vi "Example_HVI_TDC_DualHistograms.vi"() -> ()   [LabVIEW 2013]
panel:
  out "VI Path":string
  out "cycle Count":i32
  out "Waiting HVI...":i32
  out "Var10=>\nHVIrunning":i32
  in  "Number variable\nHVI runinng":i32=10
  out "Get HVI-Module Status":errorcluster
  out "HVI open Status":errorcluster
  out "errorOut HistogramRead":errorcluster
  in  "bins":i32=50 min=0 max=990 step=10
  out "Histogram":u32[](graph)
  out "histogramOut":u32[](array[numeric])
  in  "Finish Program":bool
  out "Histogram 1 PeakBin":i32
  out "Histogram 1 Peak":i32
  out "Histogram 0 PeakBin":i32
  out "Histogram 0 Peak":i32
  out "Ch1 RateCounter":i32
  out "Ch0 RateCounter":i32
  in  "Number variable \nHistogram 1 PeakBin":i32=5
  in  "Number variable\nHistogram 1 Peak":i32=4
  in  "Number variable \nHistogram 0 PeakBin":i32=3
  in  "Number variable \nHistogram 0 Peak":i32=2
  in  "Name variable \nCh1 RateCounter":string="Variable 1"
  in  "Name variable  \nCh0 RateCounter":string="Variable 0"
  in  "Module name in HVI":string="TDC"
  out "HVIIDOut":i32
  out "moduleIDOut":i32
  out "Close HVI Status":errorcluster
  in  "HVI file":string=".\\Example_HVI_TDC_DualHistograms.HVI"
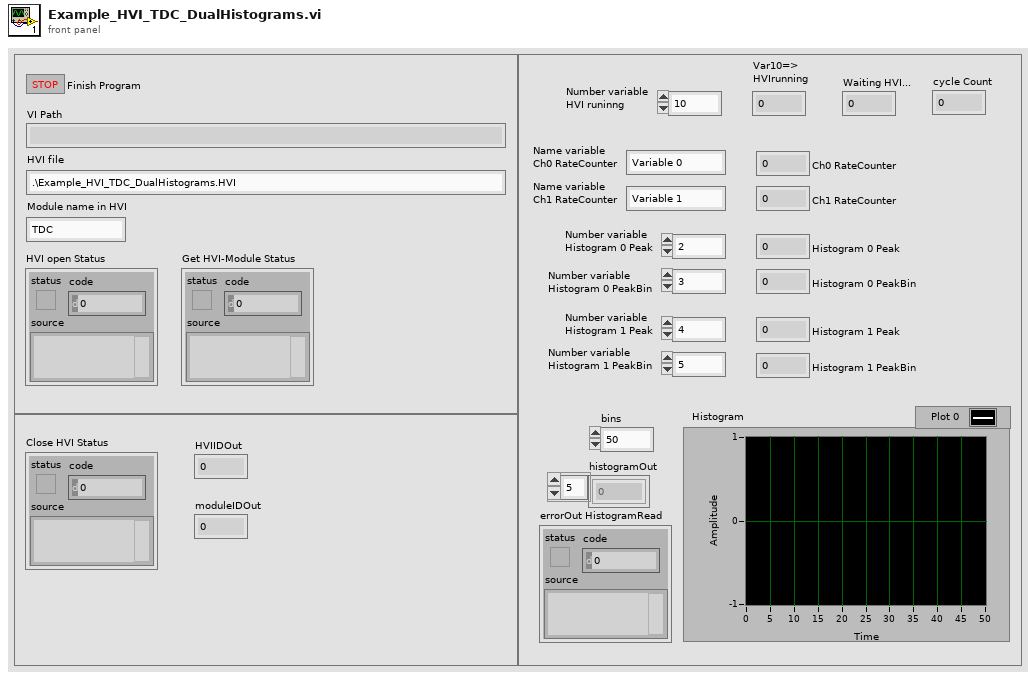
[diagram p1: front panel]
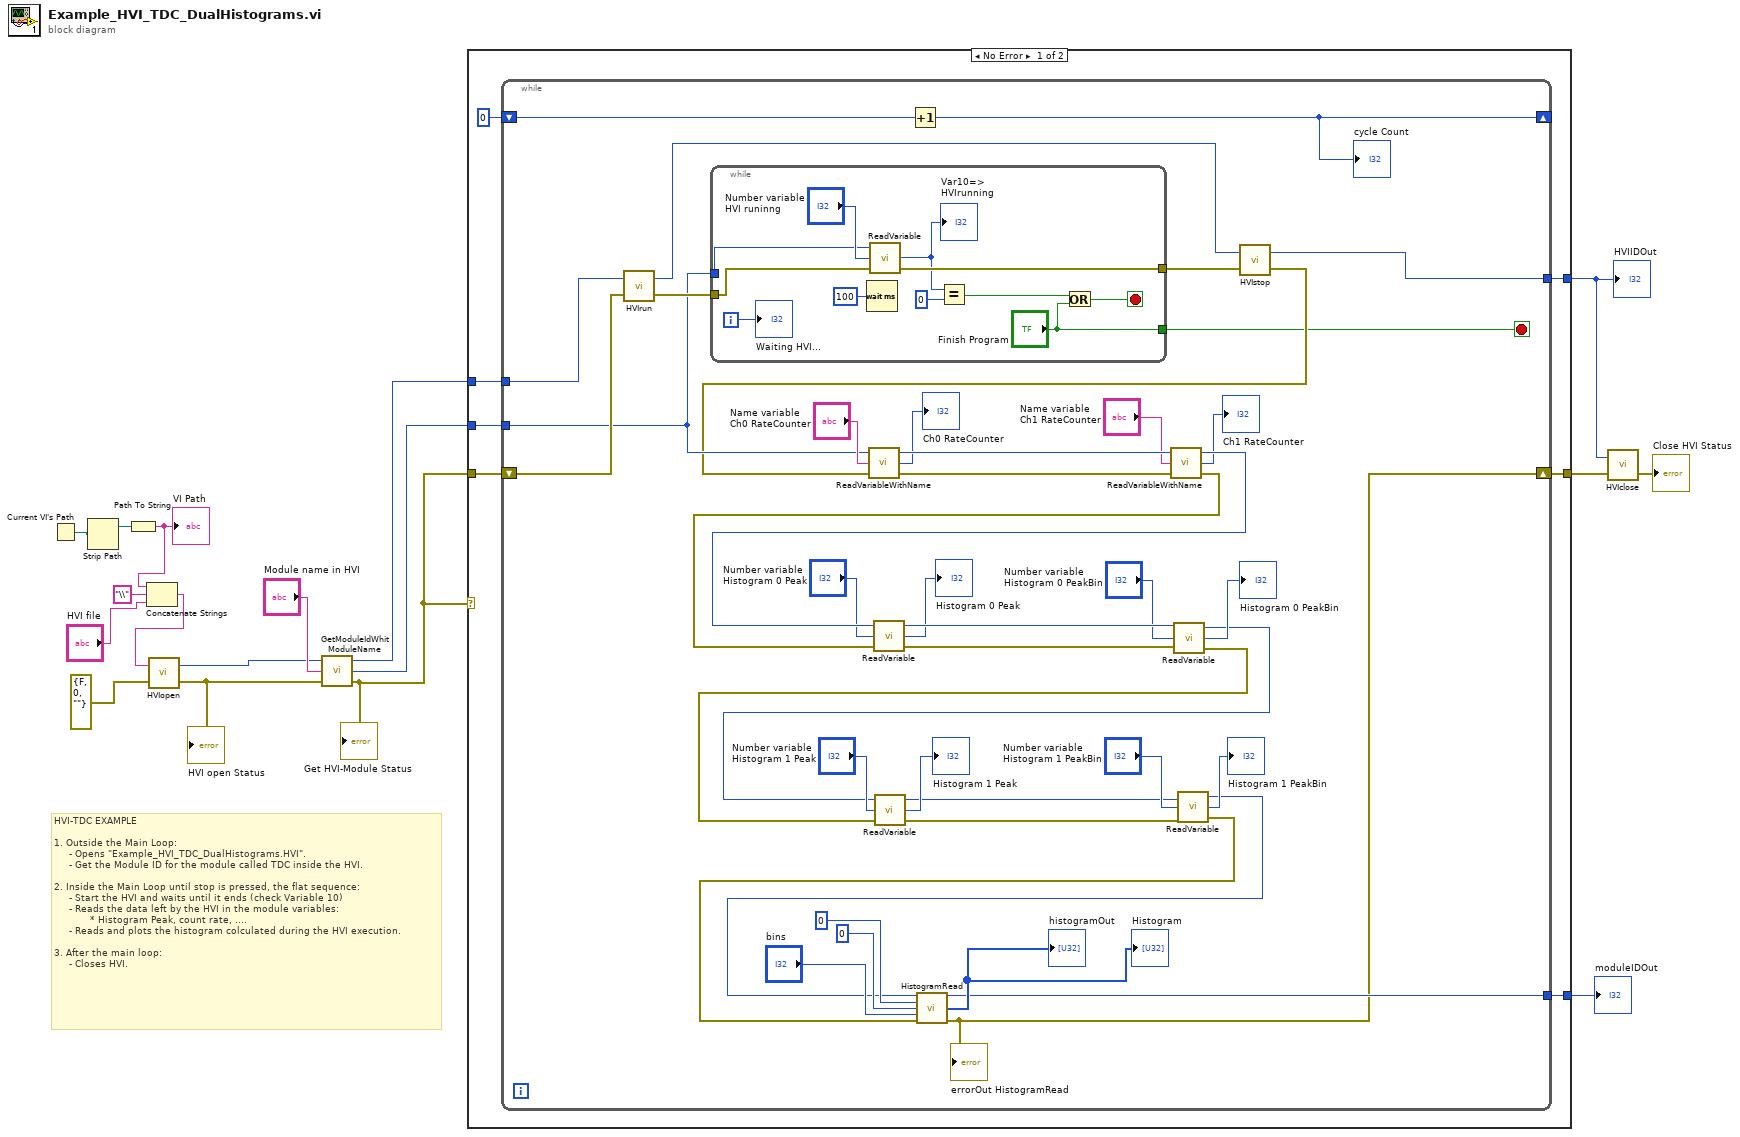
[diagram p0: block diagram]
diagram:
  # "HVI-TDC EXAMPLE\n\n1. Outside the Main Loop:\n     - Opens \"Example_HVI_TDC_DualHistograms.HVI\".\n     - Get the Module ID for the module called TDC inside the HVI.\n\n2. Inside the Main Loop until stop is pressed, the flat sequence:\n     - Start the HVI and waits until it ends (check Variable 10)\n     - Reads the data left by the HVI in the module variables:\n            * Histogram Peak, count rate, ....\n     - Reads and plots the histogram colculated during the HVI execution.\n\n3. After the main loop:\n     - Closes HVI."
  n1 = Current VI's Path() -> (path=w13:path)
  n2 = Strip Path(path=w13) -> (stripped path=w12:path)  [unwired: 1 out]
  n3 = Path To String(path=w12) -> (string=w11:string)
  "VI Path" <- w11
  n4 = Concatenate Strings(w11, "\\" ("string"), "HVI file") -> (w8:string)
  n5 = call <vilib>:"HVIopen.vi"("errorIn"=errorcluster {"status"=FALSE, "code"=0, "source"=""}, "HVIfile"=w8) -> ("errorOut"=w6:errorcluster, "HVIID"=w5:i32)
  "HVI open Status" <- w6
  n6 = call <vilib>:"GetModuleIdWhitModuleName.vi"("errorIn"=w6, "ModuleName"="Module name in HVI", "HVIID"=w5) -> ("errorOut"=w1:errorcluster, "ModuleID"=w16:u32, "HVIIDOut"=w15:i32)
  "Get HVI-Module Status" <- w1
  n7 = case shown="No Error" w1 {
    tunnel: w16 -> [w24 w77]
    tunnel: w1 -> [w23 w78]
    tunnel: w15 -> [w22 w79]
    tunnel: [w21 w77] -> w14
    tunnel: [w19 w79] -> w3
    tunnel: [w18 w78] -> w2
    frame No Error {
      n8 = while {
        tunnel: w24 -> [w31]
        tunnel: w22 -> [w37]
        tunnel: [w35] -> w21
        shift-right: [w29] -> w18
        shift-left: w23 -> [w36]
        tunnel: [w28] -> w19
        shift-right: [w25] -> _
        shift-left: 0 ("x") -> [w26]
        stop <- w27 stop-if-true
        n9 = call <vilib>:"HVIrun.vi"("errorIn"=w36, "HVIID"=w37) -> ("errorOut"=w33:errorcluster, "HVIIDOut"=w34:i32)
        n10 = while {
          tunnel: w33 -> [w75]
          tunnel: [w74] -> w32
          tunnel: w31 -> [w73]
          tunnel: ["Finish Program"] -> w27
          i -> [w70]
          stop <- w67 stop-if-true
          n11 = Wait (ms)(milliseconds to wait=u32 100) -> ()  [unwired: 1 out]
          n12 = call <vilib>:"ReadVariable.vi"("errorIn"=w75, "Number"="Number variable\nHVI runinng", "ModuleID"=w73) -> ("errorOut"=w74:errorcluster, "variableValue"=w72:i32)  [unwired: 1 out]
          "Var10=>\nHVIrunning" <- w72
          n13 = Equal?(x=w72, y=0) -> (x = y?=w68:bool)
          n14 = Or(x=w68, y="Finish Program") -> (x .or. y?=w67:bool)
          "Waiting HVI..." <- w70
        }
        n15 = Increment(x=w26) -> (x+1=w25:i32)
        "cycle Count" <- w25
        n16 = call <vilib>:"HVIstop.vi"("errorIn"=w32, "HVIID"=w34) -> ("errorOut"=w30:errorcluster, "HVIIDOut"=w28:i32)
        n17 = call <vilib>:"ReadVariableWithName.vi"("errorIn"=w30, "Name"="Name variable  \nCh0 RateCounter", "ModuleID"=w31) -> ("errorOut"=w65:errorcluster, "variableValue"=→"Ch0 RateCounter":i32, "ModuleIDOut"=w61:i32)
        n18 = call <vilib>:"ReadVariableWithName.vi"("errorIn"=w65, "Name"="Name variable \nCh1 RateCounter", "ModuleID"=w61) -> ("errorOut"=w64:errorcluster, "variableValue"=→"Ch1 RateCounter":i32, "ModuleIDOut"=w60:i32)
        n19 = call <vilib>:"ReadVariable.vi"("errorIn"=w64, "Number"="Number variable \nHistogram 0 Peak", "ModuleID"=w60) -> ("errorOut"=w63:errorcluster, "variableValue"=→"Histogram 0 Peak":i32, "ModuleIDOut"=w59:i32)
        n20 = call <vilib>:"ReadVariable.vi"("errorIn"=w63, "Number"="Number variable \nHistogram 0 PeakBin", "ModuleID"=w59) -> ("errorOut"=w40:errorcluster, "variableValue"=→"Histogram 0 PeakBin":i32, "ModuleIDOut"=w45:i32)
        n21 = call <vilib>:"ReadVariable.vi"("errorIn"=w40, "Number"="Number variable\nHistogram 1 Peak", "ModuleID"=w45) -> ("errorOut"=w62:errorcluster, "variableValue"=→"Histogram 1 Peak":i32, "ModuleIDOut"=w46:i32)
        n22 = call <vilib>:"ReadVariable.vi"("errorIn"=w62, "Number"="Number variable \nHistogram 1 PeakBin", "ModuleID"=w46) -> ("errorOut"=w38:errorcluster, "variableValue"=→"Histogram 1 PeakBin":i32, "ModuleIDOut"=w39:i32)
        n23 = call <vilib>:"HistogramRead.vi"("moduleID"=w39, "nHistogram"=0, "startBin"=0, "nBins"="bins", "errorIn"=w38) -> ("moduleIDout"=w35:i32, "histogramData"=→"histogramOut" →"Histogram":u32[], "errorOut"=w29:errorcluster)  [unwired: 8 in]
        "errorOut HistogramRead" <- w29
      }
    }
    frame Error {
    }
  }
  "moduleIDOut" <- w14
  "HVIIDOut" <- w3
  n24 = call <vilib>:"HVIclose.vi"("errorIn"=w2, "HVIID"=w3) -> ("errorOut"=→"Close HVI Status":errorcluster)  [unwired: 1 in]
